vi "VCS Halt Position Movement.vi"(8 "error in (no error)":errorcluster, 11 "axis in":cluster{"keyHandle":u32, "nodeId":u16}={"keyHandle"=0, "nodeId"=1}) -> (0 "error out":errorcluster, 3 "axis out":cluster{"keyHandle":u32, "nodeId":u16}={"keyHandle"=0, "nodeId"=1})   [LabVIEW 2019, in "maxonEPOS.lvlib"]
doc: "With function <B>VCS Halt Position Movement</B> movement stops with profile deceleration."
uses:
  Examples/maxonEPOS.lvlib
  Resources/EposCmd.dll
  Resources/EposCmd64.dll
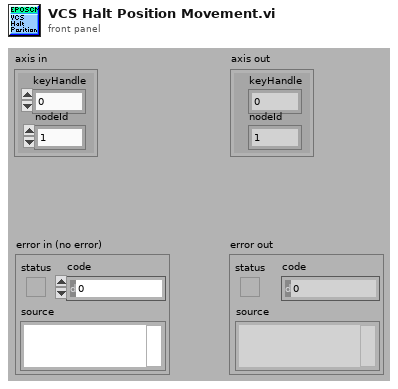
[diagram p1: front panel]
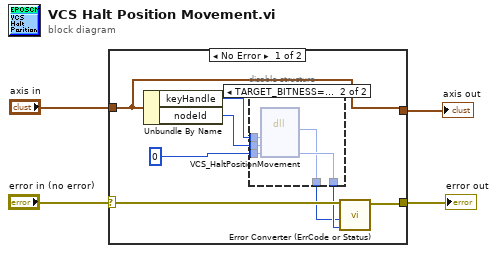
[diagram p0: block diagram]
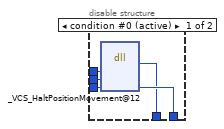
[diagram p2: hidden frame]
diagram:
  n1 = case shown="No Error" "error in (no error)" {
    selector: "error in (no error)" -> [w12 w24]
    tunnel: [w11 w24] -> w3
    tunnel: "axis in" -> [w5 w23]
    tunnel: [w5 w23] -> w1
    frame No Error {
      n2 = Unbundle By Name(w5) -> ("keyHandle"=w8:u32, "nodeId"=w7:u16)
      n3 = disable-structure shown="TARGET_BITNESS==64" {
        disable-tunnel: [w17 w22] -> w10
        disable-tunnel: [w16 w21] -> w9
        disable-tunnel: w8 -> [w15 w20]
        disable-tunnel: w7 -> [w14 w19]
        disable-tunnel: u32 0 ("pErrorCode") -> [w13 w18]
        frame condition #0 (active) {
          n4 = dll-call lib="C:/workspace/project/scancon/sw/SSI_Tool/InstrumentsInterfaces/Motordriver/maxon EPOS/Resources/EposCmd.*" fn="_VCS_HaltPositionMovement@12"("KeyHandle"=w15, "NodeId"=w14, "pErrorCode"=w13) -> (w16:i32, "pErrorCode"=w17:u32)  [unwired: 5 in, 2 out]
        }
        frame condition #1 {
          n5 = dll-call lib="C:/Sources/LabView/maxon EPOS/Resources/EposCmd64.*" fn="VCS_HaltPositionMovement" ("EposCmd.dll:_VCS_HaltPositionMovement@12")("KeyHandle"=w20, "NodeId"=w19, "pErrorCode"=w18) -> ("Rückgabetyp"=w21:i32, "pErrorCode"=w22:u32)  [unwired: 5 in, 2 out]
        }
      }
      n6 = call "Error Converter (ErrCode or Status).vi"("error code"=w10, "return type"=w9, "error in (no error)"=w12) -> ("error out"=w11:errorcluster)  [unwired: 7 in]
    }
    frame Error {
    }
  }
  "error out" <- w3
  "axis out" <- w1
